vi "CRYKernel estimation.vi"(9 "free or diffuse":bool=TRUE, 10 "Ti-11":dbl[](array[numeric]), 11 "LE":dbl[](array[numeric])) -> (3 "Kern":dbl[](array[numeric]))   [LabVIEW 2013]
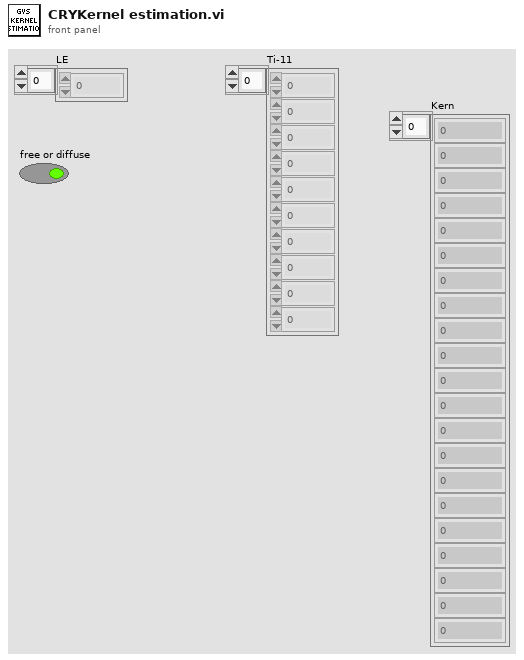
[diagram p1: front panel]
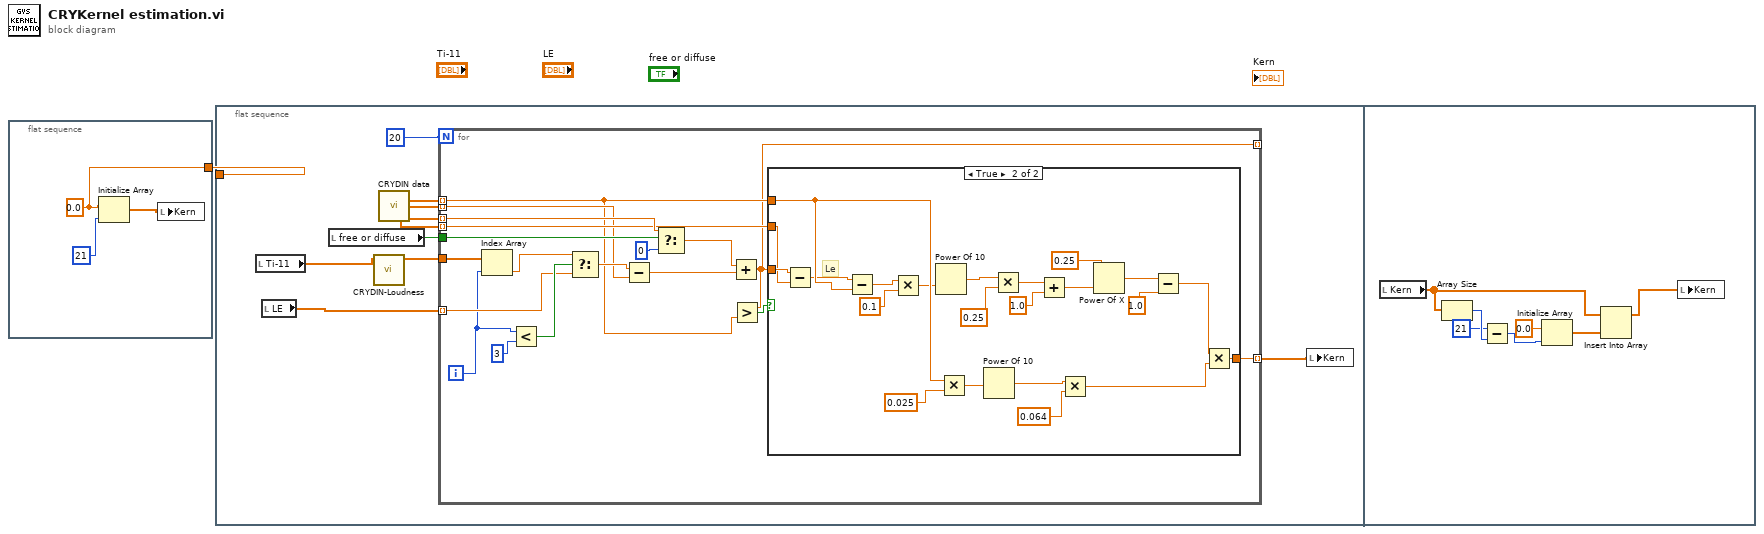
[diagram p0: block diagram]
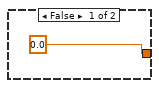
[diagram p2: hidden frame]
diagram:
  n1 = flat-sequence {
    tunnel: [w3] -> w1
    frame #0 {
      w3 = 0.0
      n2 = Initialize Array(w3, 21) -> (w2:dbl[])
      n3 = local write "Kern"(w2) -> ()
    }
  }
  n4 = flat-sequence {
    tunnel: w1 -> [_]
    frame #0 {
      n5 = local read "Ti-11"() -> (w5:dbl[])
      n6 = local read "LE"() -> (w6:dbl[])
      n7 = local read "free or diffuse"() -> (w13:bool)
      n8 = call "CRYDIN-Loudness.vi"("Ti-1"=w5) -> ("Ti"=w12:dbl[])  [unwired: 9 in]
      n9 = call "CRYDIN data.vi"() -> ("thresholdin quiet1"=w11:dbl[], "OutEar Transmission1"=w10:dbl[], "CriticalBandCorrection1"=w8:dbl[], "diffuseFieldCorrection1"=w9:dbl[])  [unwired: 8 in, 4 out]
      n10 = for {
        N: 20 -> [_]
        tunnel: w6 -> [w30] mode=indexing
        tunnel: w12 -> [w21]
        tunnel: w10 -> [w18] mode=indexing
        tunnel: w13 -> [w28]
        tunnel: w9 -> [w26] mode=indexing
        tunnel: w8 -> [w24] mode=indexing
        tunnel: w11 -> [w17] mode=indexing
        tunnel: [w23] -> w7 mode=indexing
        tunnel: [w15] -> _ mode=indexing
        i -> [w22]
        n11 = Index Array(array=w21, index=w22) -> (element=w20:dbl)
        n12 = Less?(x=w22, y=3) -> (x < y?=w31:bool)
        n13 = Select(t=w20, s=w31, f=w30) -> (s? t:f=w29:dbl)
        n14 = Subtract(x=w29, y=w18) -> (x-y=w16:dbl)
        n15 = Select(t=w26, s=w28, f=0) -> (s? t:f=w27:dbl)
        n16 = Add(x=w27, y=w16) -> (x+y=w15:dbl)
        n17 = Greater?(x=w15, y=w17) -> (0:w19:bool)
        n18 = case shown="True" w19 {
          tunnel: w15 -> [_ w55]
          tunnel: w24 -> [_ w54]
          tunnel: w17 -> [_ w49]
          tunnel: [0.0 w36] -> w23
          frame False {
          }
          frame True {
            # "Le"
            n19 = Subtract(x=w55, y=w54) -> (x-y=w34:dbl)
            n20 = Subtract(x=w34, y=w49) -> (x-y=w35:dbl)
            n21 = Multiply(x=w35, y=0.1) -> (x*y=w47:dbl)
            n22 = Power Of 10(x=w47) -> (10^x=w46:dbl)
            n23 = Multiply(x=w49, y=0.025) -> (x*y=w52:dbl)
            n24 = Power Of 10(x=w52) -> (10^x=w51:dbl)
            n25 = Multiply(x=w46, y=0.25) -> (x*y=w44:dbl)
            n26 = Add(x=w44, y=1.0) -> (x+y=w42:dbl)
            n27 = Multiply(x=w51, y=0.064) -> (x*y=w37:dbl)
            n28 = Power Of X(1:w42, 2:0.25) -> (0:w40:dbl)
            n29 = Subtract(x=w40, y=1.0) -> (x-y=w38:dbl)
            n30 = Multiply(x=w38, y=w37) -> (x*y=w36:dbl)
          }
        }
      }
      n31 = local write "Kern"(w7) -> ()
    }
    frame #1 {
      n32 = local read "Kern"() -> (w57:dbl[])
      n33 = Array Size(array=w57) -> (size(s)=w62:i32)
      n34 = Subtract(x=21, y=w62) -> (x-y=w59:i32)
      n35 = Initialize Array(0.0 ("element"), w59) -> (w58:dbl[])
      n36 = Insert Into Array(array=w57, new element=w58) -> (w56:dbl[])  [unwired: 1 in]
      n37 = local write "Kern"(w56) -> ()
    }
  }
